vi "Initialize.vi"(0 "Channel in":refnum<class "Channel.lvclass">, 1 "Calibration folder":path, 2 "Local folder":path, 3 "Fs (Hz)":dbl, 4 "Npts":i32, 5 "error in (no error)":errorcluster, 6 "SigMan Name":string, 7 "Vmax":dbl, 9 "Number":i32, 11 "Rig":string) -> (14 "Channel out":refnum<class "Channel.lvclass">, 19 "error out":errorcluster)   [LabVIEW 2020, in "Channel.lvclass"]
uses:
  Channel.lvclass
  Channel.lvclass/Channel.ctl
  Level/Level.lvclass
  Gate/Gate.lvclass
  Waveforms/Waveform/Waveform.lvclass
  Modulations/AM/AM.lvclass
  c70c4250-3272-4fce-b2d1-a2080d667a44.vi
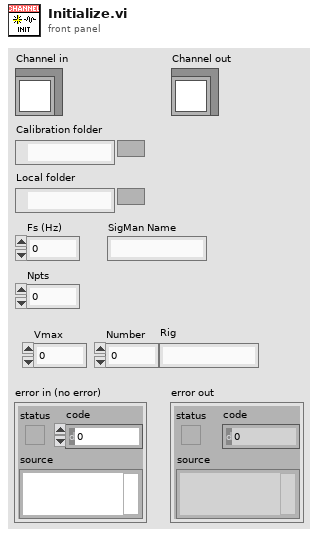
[diagram p1: front panel]
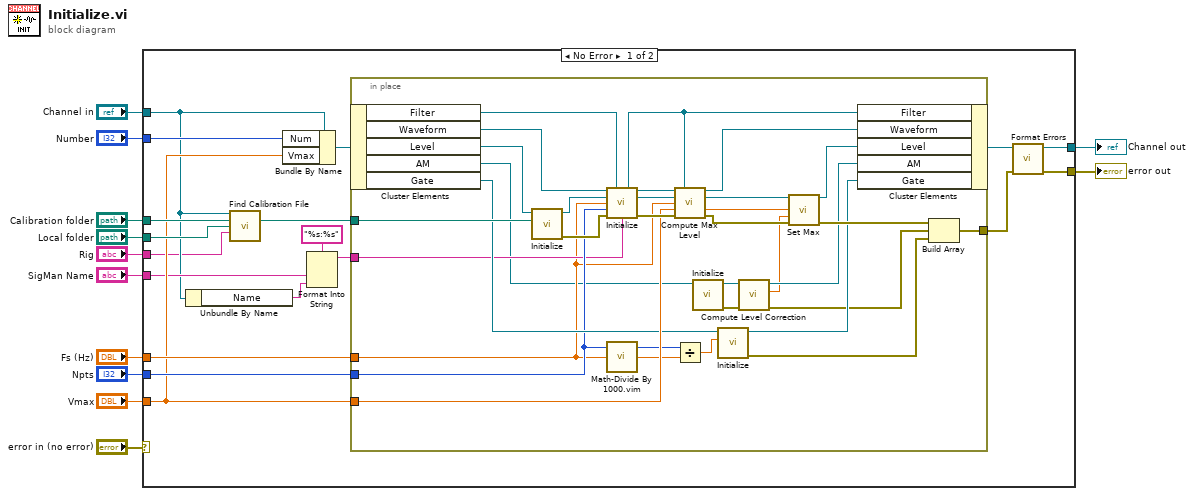
[diagram p0: block diagram]
diagram:
  n1 = case shown="No Error" "error in (no error)" {
    selector: "error in (no error)" -> [_ w64]
    tunnel: [w25 w64] -> w11
    tunnel: [w27 w63] -> w9
    tunnel: "Channel in" -> [w16 w63]
    tunnel: "Number" -> [w30 _]
    tunnel: "Fs (Hz)" -> [w24 _]
    tunnel: "Npts" -> [w23 _]
    tunnel: "Calibration folder" -> [w22 _]
    tunnel: "Local folder" -> [w21 _]
    tunnel: "Vmax" -> [w19 _]
    tunnel: "SigMan Name" -> [w17 _]
    tunnel: "Rig" -> [w13 _]
    frame No Error {
      n2 = Unbundle By Name(w16) -> ("Name"=w15:string)
      n3 = call "Find Calibration File.vi"("Channel in"=w16, "Calibration folder"=w22, "Local folder"=w21, "Rig"=w13) -> ("Calibration File"=w20:path)  [unwired: 9 in, 2 out]
      n4 = Bundle By Name(cluster=w16, "Num"=w30, "Vmax"=w19) -> (w29:refnum<class "Channel.lvclass">)
      n5 = Format Into String(format string="%s:%s", w17, w15) -> (resulting string=w14:string)  [unwired: 2 in, 1 out]
      n6 = in-place {
        in-place-border: w20 -> [w61]
        in-place-border: [w59] -> w26
        in-place-border: w24 -> [w37]
        in-place-border: w23 -> [w43]
        in-place-border: w19 -> [w52]
        in-place-border: w14 -> [w39]
        n7 = in-place-cluster #1(w29) -> ("Filter"=w40:refnum<class "Filter.lvclass">, "Waveform"=w60:refnum<class "Waveform.lvclass">, "Level"=w62:refnum<class "Level.lvclass">, "AM"=w36:refnum<class "AM.lvclass">, "Gate"=w46:refnum<class "Gate.lvclass">)
        n8 = call "Initialize.vi"("Cal file"=w61, "Level in"=w62) -> ("error out"=w53:errorcluster, "Level out"=w55:refnum<class "Level.lvclass">)  [unwired: 8 in]
        n9 = call-dynamic "Initialize.vi"("Waveform in"=w60, "Filter in"=w40, "Level in"=w55, "Fs (Hz)"=w37, "Npts"=w43, "error in (no error)"=w53, "Channel Name"=w39) -> ("Filter out"=w38:refnum<class "Filter.lvclass">, "Waveform out"=w58:refnum<class "Waveform.lvclass">, "Level out"=w54:refnum<class "Level.lvclass">, "error out"=w57:errorcluster)  [unwired: 5 in]
        n10 = call "Math-Divide By 1000.vim"("X"=w37) -> ("1000X"=w42:dbl)
        n11 = call-dynamic "Compute Max Level.vi"("Waveform in"=w58, "Filter in"=w38, "Level in"=w54, "Fs (Hz)"=w37, "Vmax"=w52, "error in (no error)"=w57) -> ("Waveform out"=w56:refnum<class "Waveform.lvclass">, "Level thru"=w50:refnum<class "Level.lvclass">, "Lmax"=w49:dbl, "error out"=w51:errorcluster)  [unwired: 6 in]
        n12 = Divide(x=w43, y=w42) -> (x/y=w41:dbl)
        n13 = call-dynamic "Initialize.vi"("AM in"=w36) -> ("error out"=w33:errorcluster, "AM out"=w35:refnum<class "AM.lvclass">)  [unwired: 9 in]
        n14 = call "Initialize.vi"("Interval (ms)"=w41, "Gate in"=w46) -> ("error out"=w44:errorcluster, "Gate out"=w45:refnum<class "Gate.lvclass">)  [unwired: 8 in]
        n15 = call "Compute Level Correction.vi"("error in (no error)"=w33, "AM in"=w35) -> ("error out"=w32:errorcluster, "Correction"=w31:dbl, "AM out"=w34:refnum<class "AM.lvclass">)  [unwired: 7 in]
        n16 = call "Set Max.vi"("Level in"=w50, "Max"=w49, "mod corr (dB)"=w31, "error in (no error)"=w51) -> ("Level out"=w48:refnum<class "Level.lvclass">, "error out"=w47:errorcluster)  [unwired: 10 in]
        n17 = in-place-cluster #1("Filter"=w38, "Waveform"=w56, "Level"=w48, "AM"=w34, "Gate"=w45) -> (w28:refnum<class "Channel.lvclass">)
        n18 = Build Array(w47, w32, w44) -> (w59:errorcluster[])
      }
      n19 = call "Format Errors.vi"("error in (no error)"=w26, "Channel in"=w28) -> ("error out"=w25:errorcluster, "Channel out"=w27:refnum<class "Channel.lvclass">)  [unwired: 8 in]
    }
    frame Error {
    }
  }
  "error out" <- w11
  "Channel out" <- w9
